vi "Enqueue Stop Message.vi"(8 "Error in":errorcluster, 11 "Queue Data":T1) -> (0 "Error out":errorcluster)   [LabVIEW 2018, in "Queue Messaging.lvlib"]
uses:
  Queue Messaging.lvlib
  QMH Template/Type Defs/EventsAndQueues--cluster.ctl
  Type Defs/Queue Message--cluster.ctl
  Event Messaging/Type Defs/Event Message--cluster.ctl
  QMH/QMH CORE.lvlib
  Event Messaging/Event Messaging.lvlib
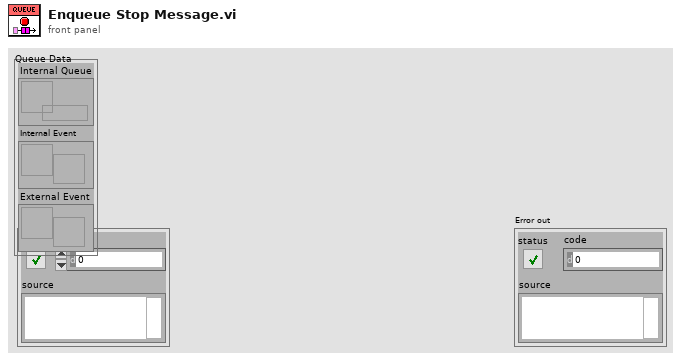
[diagram p1: front panel]
types:
  T1 = typedef "QMH CORE.lvlib/EventsAndQueues--cluster.ctl" = cluster{"Internal Queue":refnum<queue>, "Internal Event":refnum<user-event>, "External Event":refnum<user-event>}
  T2 = typedef "Queue Messaging.lvlib/Queue Message--cluster.ctl" = cluster{"Cmd":string, "Data":variant}
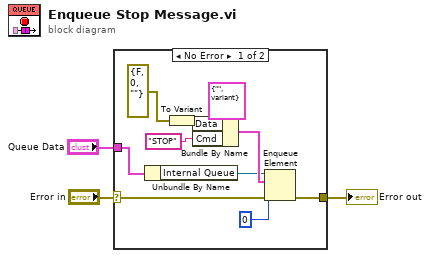
[diagram p0: block diagram]
diagram:
  n1 = case shown="No Error" "Error in" {
    selector: "Error in" -> [w9 w14]
    tunnel: "Queue Data" -> [w11 _]
    tunnel: [w8 w14] -> w2
    frame No Error {
      n2 = Unbundle By Name(w11) -> ("Internal Queue"=w7:refnum<queue>)
      n3 = To Variant(anything=errorcluster {"status"=FALSE, "code"=0, "source"=""} ("error constant")) -> (Variant=w4:variant)
      n4 = Bundle By Name(cluster=T2 {"Cmd"="", "Data"=variant} ("Message"), "Data"=w4, "Cmd"="STOP") -> (w12:T2)
      n5 = Enqueue Element(queue=w7, element=w12, timeout in ms (-1)=0, error in (no error)=w9) -> (error out=w8:errorcluster)  [unwired: 2 out]
    }
    frame Error {
    }
  }
  "Error out" <- w2
